vi "Set_Osc_Conf_L1.vi"(0 "VISA resource name":refnum<visa-resource-name>="Oscilloscope", 1 "Amplitude IN":dbl=0.25, 2 "Trigger Level IN":dbl=1.65, 3 "Pulse Width in seconds IN":dbl=2.5e-09, 4 "Position 1":dbl, 5 "error in (no error)":errorcluster, 6 "Channel 1":bool=TRUE, 7 "Channel 3":bool=TRUE, 8 "Channel 2":bool=TRUE, 9 "Channel 4":bool=TRUE) -> (14 "VISA resource name out":refnum<visa-resource-name>="Oscilloscope", 19 "error out":errorcluster)   [LabVIEW 2012]
uses:
  C/Program Files/National Instruments/LabVIEW 2012/instr.lib/Agilent 8000 Series/Public/Configure/Configure Trigger (Edge).vi
  <instrlib>/Agilent 8000 Series/Public/Configure/Configure Math (Binary Operation).vi
  <instrlib>/Agilent 8000 Series/Agilent 8000 Series.lvlib
panel:
  in  "Channel 4":i32(ring)=4 items=["Channel 1"=1, "Channel 2"=2, "Channel 3"=3, "Channel 4"=4]
  in  "Vertical Coupling 4":i32(ring)=1 items=["AC", "DC"]
  in  "Probe Attenuation 4":dbl=1.0
  in  "Vertical Range Scaler 4":dbl=2.0
  in  "Vertical Offset 4":dbl
  in  "Input Impedance 4":u32(ring) items=["50 ohms", "1 Mohms"]
  in  "Channel 3":i32(ring)=3 items=["Channel 1"=1, "Channel 2"=2, "Channel 3"=3, "Channel 4"=4]
  in  "Vertical Coupling 3":i32(ring)=1 items=["AC", "DC"]
  in  "Probe Attenuation 3":dbl=1.0
  in  "Vertical Range Scaler 3":dbl=2.0
  in  "Vertical Offset 3":dbl
  in  "Input Impedance 3":u32(ring) items=["50 ohms", "1 Mohms"]
  in  "Channel 2":i32(ring)=2 items=["Channel 1"=1, "Channel 2"=2, "Channel 3"=3, "Channel 4"=4]
  in  "Vertical Coupling 2":i32(ring)=1 items=["AC", "DC"]
  in  "Probe Attenuation 2":dbl=1.0
  in  "Vertical Range Scaler 2":dbl=2.0
  in  "Vertical Offset 2":dbl
  in  "Input Impedance 2":u32(ring) items=["50 ohms", "1 Mohms"]
  in  "Trigger Coupling":u16(ring)=1 items=["AC", "DC", "Low Freq Reject", "High Freq Reject"]
  in  "Trigger Slope":u16(ring) items=["Positive", "Negative"]
  in  "Trigger Source":i32(ring)=1 items=["Channel 1"=1, "Channel 2"=2, "Channel 3"=3, "Channel 4"=4, "Digital 0"=13, "Digital 1"=14, "Digital 2"=15, "Digital 3"=16, "Digital 4"=17, "Digital 5"=18, "Digital 6"=19, "Digital 7"=20, "Digital 8"=21, "Digital 9"=22, "Digital 10"=23, "Digital 11"=24, "Digital 12"=25, "Digital 13"=26, "Digital 14"=27, "Digital 15"=28, "Aux"=29, "Line"=30]
  in  "Timebase Scaler":dbl=10.0
  in  "Record Length":i32=5000
  in  "Input Impedance 1":u32(ring) items=["50 ohms", "1 Mohms"]
  in  "Vertical Offset 1":dbl
  in  "Vertical Range Scaler 1":dbl=2.0
  in  "Probe Attenuation 1":dbl=1.0
  in  "Vertical Coupling 1":i32(ring)=1 items=["AC", "DC"]
  in  "Channel 1":i32(ring)=1 items=["Channel 1"=1, "Channel 2"=2, "Channel 3"=3, "Channel 4"=4]
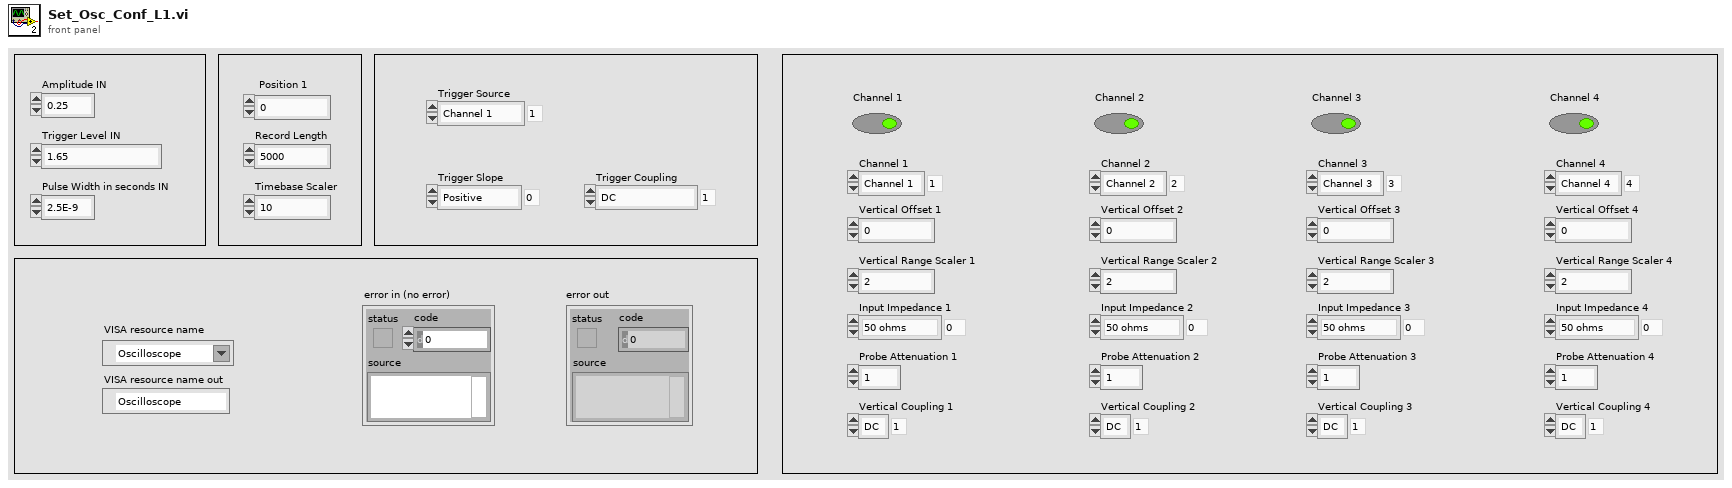
[diagram p1: front panel]
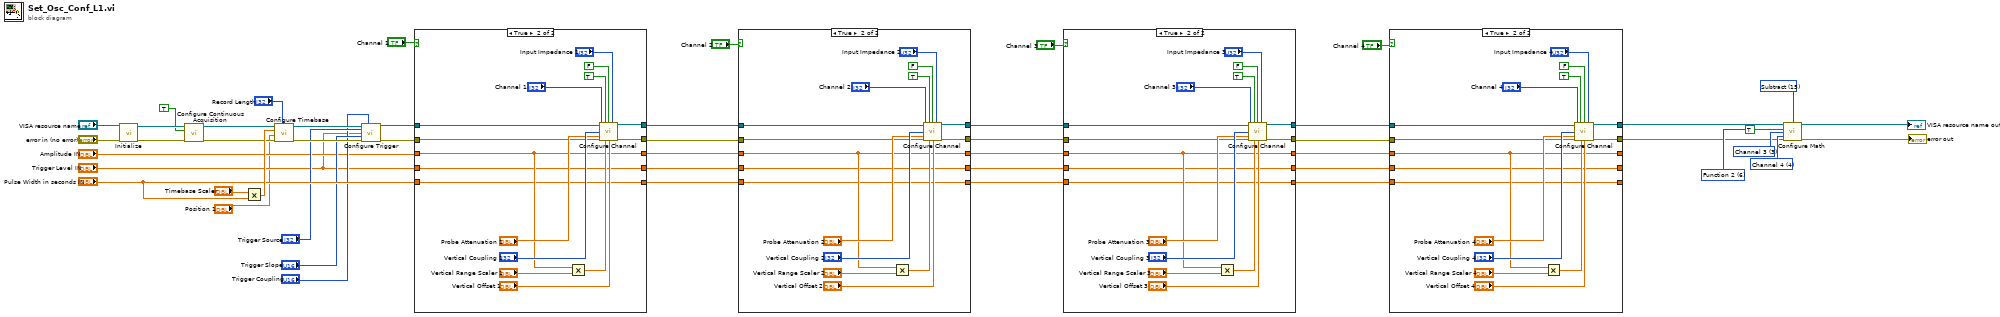
[diagram p0: block diagram]
diagram:
  w5 = u16 6 items=["Function 1"=5, "Function 2"=6, "Function 3"=7, "Function 4"=8] ("Math Channel (5: Function 1)")
  w6 = u16 15 items=["Add"=12, "Divide"=13, "Multiply"=14, "Subtract"=15, "Common Mode"=16, "Versus"=17] ("Math Operation (12: Add)")
  w8 = 3 items=["Channel 1"=1, "Channel 2"=2, "Channel 3"=3, "Channel 4"=4] ("Channel (1: Channel 1)")
  w7 = 4 items=["Channel 1"=1, "Channel 2"=2, "Channel 3"=3, "Channel 4"=4] ("Channel (1: Channel 1)")
  n1 = call <instrlib>:"Initialize.vi"("error in (no error)"="error in (no error)", "VISA resource name"="VISA resource name") -> ("error out"=w12:errorcluster, "VISA resource name out"=w15:refnum<visa-resource-name>)  [unwired: 8 in]
  n2 = call <instrlib>:"Configure Continuous Acquisition.vi"("error in (no error)"=w12, "Enable Continuous Acquisition Mode (T:Enable)"=TRUE, "VISA resource name"=w15) -> ("error out"=w13:errorcluster, "VISA resource name out"=w14:refnum<visa-resource-name>)  [unwired: 7 in]
  n3 = Multiply(x="Timebase Scaler", y="Pulse Width in seconds IN") -> (x*y=w44:dbl)
  n4 = call "Configure Timebase.vi"("Record Length (1000)"="Record Length", "error in (no error)"=w13, "Position (0.0 s)"="Position 1", "Timebase (0.005 s)"=w44, "VISA resource name"=w14) -> ("error out"=w40:errorcluster, "VISA resource name out"=w42:refnum<visa-resource-name>)  [unwired: 5 in]
  n5 = call-poly "Configure Trigger.vi"("VISA resource name"=w42, "Trigger Coupling (1 : DC)"="Trigger Coupling", "Trigger Source (1: Channel 1)"="Trigger Source", "Trigger Level (0.0 V)"="Trigger Level IN", "Trigger Slope (0: Positive)"="Trigger Slope", "error in (no error)"=w40) -> ("VISA resource name out"=w41:refnum<visa-resource-name>, "error out"=w39:errorcluster)  [unwired: 8 in]
  n6 = case shown="True" "Channel 1" {
    tunnel: w39 -> [w53 w58]
    tunnel: w41 -> [w54 w59]
    tunnel: "Amplitude IN" -> [w52 w57]
    tunnel: [w54 w61] -> w34
    tunnel: [w53 w60] -> w33
    tunnel: "Trigger Level IN" -> [w51 w56]
    tunnel: [w52 w57] -> w32
    tunnel: [w51 w56] -> w31
    tunnel: "Pulse Width in seconds IN" -> [w50 w55]
    tunnel: [w50 w55] -> w30
    frame False {
    }
    frame True {
      n7 = Multiply(x=w57, y="Vertical Range Scaler 1") -> (x*y=w65:dbl)
      n8 = call <instrlib>:"Configure Channel.vi"("VISA resource name"=w59, "Enable Channel (Enable)"=TRUE, "BW Limit 20MHz (Disable)"=FALSE, "Input Impedance (1: 1 Mohms)"="Input Impedance 1", "Channel (1: Channel 1)"="Channel 1", "Vertical Coupling (1: DC)"="Vertical Coupling 1", "Probe Attenuation (1.0)"="Probe Attenuation 1", "error in (no error)"=w58, "Vertical Range (2.0 V)"=w65, "Vertical Offset (0.0 V)"="Vertical Offset 1") -> ("VISA resource name out"=w61:refnum<visa-resource-name>, "error out"=w60:errorcluster)  [unwired: 4 in]
    }
  }
  n9 = case shown="True" "Channel 2" {
    tunnel: w33 -> [w74 w79]
    tunnel: w34 -> [w75 w80]
    tunnel: w32 -> [w73 w78]
    tunnel: [w75 w82] -> w28
    tunnel: [w74 w81] -> w27
    tunnel: w31 -> [w72 w77]
    tunnel: [w73 w78] -> w26
    tunnel: [w72 w77] -> w25
    tunnel: w30 -> [w71 w76]
    tunnel: [w71 w76] -> w24
    frame False {
    }
    frame True {
      n10 = Multiply(x=w78, y="Vertical Range Scaler 2") -> (x*y=w86:dbl)
      n11 = call <instrlib>:"Configure Channel.vi"("VISA resource name"=w80, "Enable Channel (Enable)"=TRUE, "BW Limit 20MHz (Disable)"=FALSE, "Input Impedance (1: 1 Mohms)"="Input Impedance 2", "Channel (1: Channel 1)"="Channel 2", "Vertical Coupling (1: DC)"="Vertical Coupling 2", "Probe Attenuation (1.0)"="Probe Attenuation 2", "error in (no error)"=w79, "Vertical Range (2.0 V)"=w86, "Vertical Offset (0.0 V)"="Vertical Offset 2") -> ("VISA resource name out"=w82:refnum<visa-resource-name>, "error out"=w81:errorcluster)  [unwired: 4 in]
    }
  }
  n12 = case shown="True" "Channel 3" {
    tunnel: w27 -> [w95 w100]
    tunnel: w28 -> [w96 w101]
    tunnel: w26 -> [w94 w99]
    tunnel: [w96 w103] -> w22
    tunnel: [w95 w102] -> w21
    tunnel: w25 -> [w93 w98]
    tunnel: [w94 w99] -> w20
    tunnel: [w93 w98] -> w19
    tunnel: w24 -> [w92 w97]
    tunnel: [w92 w97] -> w18
    frame False {
    }
    frame True {
      n13 = Multiply(x=w99, y="Vertical Range Scaler 3") -> (x*y=w107:dbl)
      n14 = call <instrlib>:"Configure Channel.vi"("VISA resource name"=w101, "Enable Channel (Enable)"=TRUE, "BW Limit 20MHz (Disable)"=FALSE, "Input Impedance (1: 1 Mohms)"="Input Impedance 3", "Channel (1: Channel 1)"="Channel 3", "Vertical Coupling (1: DC)"="Vertical Coupling 3", "Probe Attenuation (1.0)"="Probe Attenuation 3", "error in (no error)"=w100, "Vertical Range (2.0 V)"=w107, "Vertical Offset (0.0 V)"="Vertical Offset 3") -> ("VISA resource name out"=w103:refnum<visa-resource-name>, "error out"=w102:errorcluster)  [unwired: 4 in]
    }
  }
  n15 = case shown="True" "Channel 4" {
    tunnel: w21 -> [w116 w121]
    tunnel: w22 -> [w117 w122]
    tunnel: w20 -> [w115 w120]
    tunnel: [w117 w124] -> w3
    tunnel: [w116 w123] -> w4
    tunnel: w19 -> [w114 w119]
    tunnel: [w115 w120] -> _
    tunnel: [w114 w119] -> _
    tunnel: w18 -> [w113 w118]
    tunnel: [w113 w118] -> _
    frame False {
    }
    frame True {
      n16 = Multiply(x=w120, y="Vertical Range Scaler 4") -> (x*y=w128:dbl)
      n17 = call <instrlib>:"Configure Channel.vi"("VISA resource name"=w122, "Enable Channel (Enable)"=TRUE, "BW Limit 20MHz (Disable)"=FALSE, "Input Impedance (1: 1 Mohms)"="Input Impedance 4", "Channel (1: Channel 1)"="Channel 4", "Vertical Coupling (1: DC)"="Vertical Coupling 4", "Probe Attenuation (1.0)"="Probe Attenuation 4", "error in (no error)"=w121, "Vertical Range (2.0 V)"=w128, "Vertical Offset (0.0 V)"="Vertical Offset 4") -> ("VISA resource name out"=w124:refnum<visa-resource-name>, "error out"=w123:errorcluster)  [unwired: 4 in]
    }
  }
  n18 = call-poly <instrlib>:"Configure Math.vi"("VISA resource name"=w3, "Enable Math Channel (T:Enable)"=TRUE, "Math Operation (12: Add)"=w6, "Math Channel (5: Function 1)"=w5, "Math Operand (1: Channel 1)"=w8, "Math Operand (2: Channel 2)"=w7, "error in (no error)"=w4) -> ("VISA resource name out"=→"VISA resource name out":refnum<visa-resource-name>, "error out"=→"error out":errorcluster)  [unwired: 7 in]
